vi "PySet3.vi"(1 "Value":string, 2 "Attribute":string) -> (0 "Error":bool)   [LabVIEW 2014]
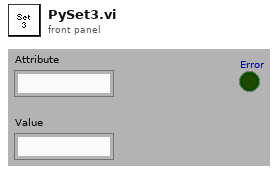
[diagram p1: front panel]
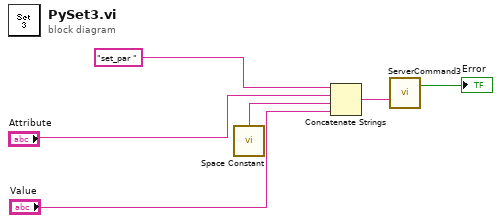
[diagram p0: block diagram]
diagram:
  n1 = call <vilib>:"Space Constant.vi"() -> ("String"=w1:string)
  n2 = Concatenate Strings("set_par " ("string"), "Attribute", w1, "Value") -> (w6:string)
  n3 = call "ServerCommand3.vi"("Command"=w6) -> ("Error"=→"Error":bool)  [unwired: 1 out]
